vi "Temperatura.vi"() -> ()   [LabVIEW 2014]
uses:
  <vilib>/LabVIEW Interface for Arduino/Type Defs/Board Type.ctl
  <vilib>/LabVIEW Interface for Arduino/LabVIEW Interface for Arduino.lvlib
panel:
  in  "Board Type":T1
  in  "VISA resource":refnum<visa-resource-name>
  out "Temperatura":dbl(slide) scale=0.0..70.0
  in  "Parar":bool
  # "Configuración"
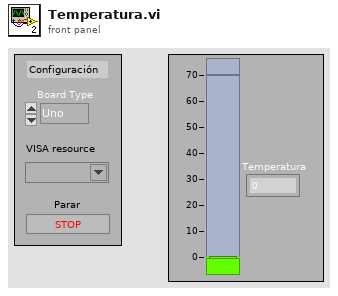
[diagram p1: front panel]
types:
  T1 = typedef "LabVIEW Interface for Arduino.lvlib/Board Type.ctl" = enum16{"Uno", "Dimuelanove w/Atmega 328", "Mega 2560"}
  T2 = typedef "LabVIEW Interface for Arduino.lvlib/Arduino Resource.ctl" = cluster{"VISA resource":refnum<visa-resource-name>, "Board Type":T1, "Connection Type":enum8{"USB / Serial"}, "Bytes Per Packet (15)":u8}
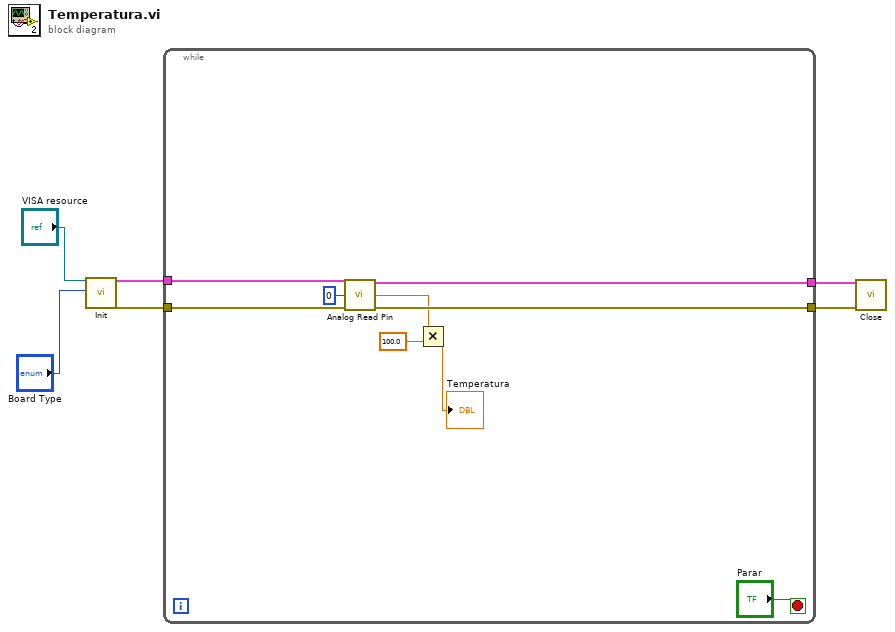
[diagram p0: block diagram]
diagram:
  n1 = call <vilib>:"Init.vi"("VISA resource"="VISA resource", "Board Type (Uno)"="Board Type") -> ("Arduino Resource"=w6:T2, "error out"=w5:errorcluster)  [unwired: 16 in]
  n2 = while {
    tunnel: w6 -> [w14]
    tunnel: w5 -> [w13]
    tunnel: [w12] -> w4
    tunnel: [w11] -> w3
    stop <- "Parar" stop-if-true
    n3 = call <vilib>:"Analog Read Pin.vi"("Arduino Resource"=w14, "Analog Input Pin (0)"=u8 0, "error in"=w13) -> ("Arduino Resource"=w12:T2, "Voltage"=w9:dbl, "error out"=w11:errorcluster)  [unwired: 10 in]
    n4 = Multiply(x=w9, y=100.0) -> (x*y=→"Temperatura":dbl)
  }
  n5 = call <vilib>:"Close.vi"("Arduino Resource"=w4, "error in"=w3) -> ()  [unwired: 13 in, 1 out]
